vi "Position Invalid Test.vi"(5 "VI reference":refnum<vi>, 7 "Centered Position":T1, 8 "error in":errorcluster, 11 "Editor Position in":refnum<class "Editor Position.lvclass">) -> (0 "error out":errorcluster, 3 "Editor Position out":refnum<class "Editor Position.lvclass">)   [LabVIEW 2020, in "Editor Position.lvclass"]
doc: "Tests the how the Set Editor Position.vi reacts to an invalid position."
uses:
  Editor Position.lvclass
  Editor Position.lvclass/Editor Position.ctl
  vi.lib/LabVIEW Icon API/lv_icon/lv_icon.lvlib
  <vilib>/Utility/miscctls.llb/LVRectTypeDef.ctl
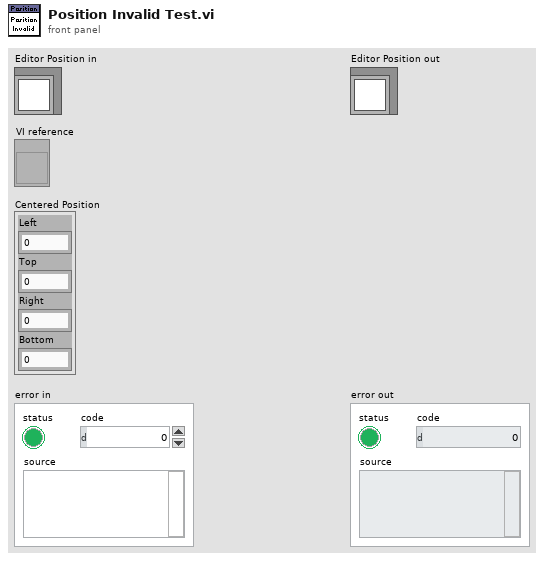
[diagram p1: front panel]
types:
  T1 = typedef "LVRectTypeDef.ctl" = cluster{"Left":i16, "Top":i16, "Right":i16, "Bottom":i16}
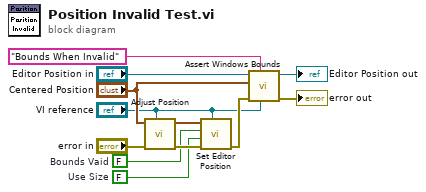
[diagram p0: block diagram]
diagram:
  w5 = FALSE  # Use Size
  w6 = FALSE  # Bounds Vaid
  n1 = call "Adjust Position.vi"("VI in"="VI reference", "error in"="error in", "Current Position"="Centered Position") -> ("error out"=w9:errorcluster, "Adjusted Position"=w4:T1)  [unwired: 7 in]
  n2 = call "Set Editor Position.vi"("IE VI Ref"="VI reference", "error in"=w9, "Use Size"=w5, "Bounds Vaid"=w6, "Window Bounds"=w4) -> ("error out"=w12:errorcluster)  [unwired: 6 in]
  n3 = call "Assert Windows Bounds.vi"("VI reference"="VI reference", "Test Description"="Bounds When Invalid" ("Description"), "error in"=w12, "Expected Position"="Centered Position", "Editor Position in"="Editor Position in") -> ("error out"=→"error out":errorcluster, "Editor Position out"=→"Editor Position out":refnum<class "Editor Position.lvclass">)  [unwired: 5 in]
